vi "Save file.vi"(0 "S1_Current":dbl[](array[numeric]), 1 "S1_Voltage":dbl[](array[numeric]), 2 "S2_Current":dbl[](array[numeric]), 3 "S2_Voltage":dbl[](array[numeric]), 4 "current time":timestamp, 5 "Save path":path, 6 "Save":bool) -> ()   [LabVIEW 2018]
uses:
  <vilib>/Utility/file.llb/Write To Spreadsheet File (string).vi
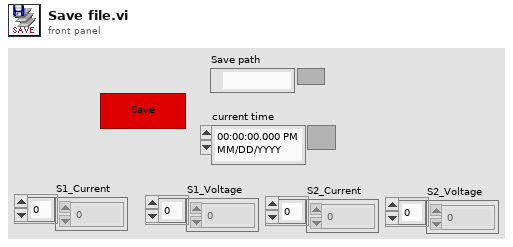
[diagram p1: front panel]
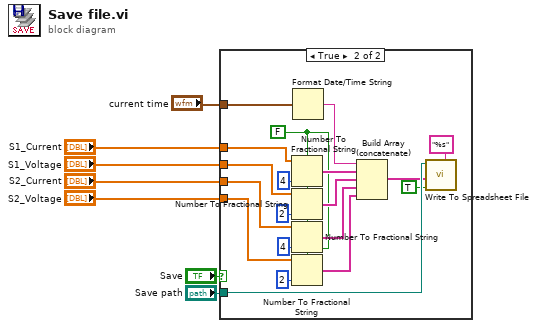
[diagram p0: block diagram]
diagram:
  n1 = case shown="True" "Save" {
    tunnel: "current time" -> [_ w25]
    tunnel: "Save path" -> [_ w12]
    tunnel: "S1_Current" -> [_ w22]
    tunnel: "S1_Voltage" -> [_ w19]
    tunnel: "S2_Current" -> [_ w16]
    tunnel: "S2_Voltage" -> [_ w15]
    frame False {
    }
    frame True {
      w10 = FALSE ("use system decimal point (T)")
      n2 = Number To Fractional String(use system decimal point (T)=w10, number=w22, precision (6)=4) -> (F-format string=w21:string[])  [unwired: 1 in]
      n3 = Number To Fractional String(use system decimal point (T)=w10, number=w19, precision (6)=2) -> (F-format string=w20:string[])  [unwired: 1 in]
      n4 = Number To Fractional String(use system decimal point (T)=w10, number=w16, precision (6)=4) -> (F-format string=w14:string[])  [unwired: 1 in]
      n5 = Number To Fractional String(use system decimal point (T)=w10, number=w15, precision (6)=2) -> (F-format string=w13:string[])  [unwired: 1 in]
      n6 = Format Date/Time String(seconds (now)=w25) -> (date/time string=w26:string)  [unwired: 2 in]
      n7 = Build Array (concatenate)(w26, w21, w20, w14, w13) -> (w11:string[])
      n8 = call-poly <vilib>:"Write To Spreadsheet File.vi"("format (%s)"="%s", "append to file? (new file:F)"=TRUE, "1D data"=w11, "file path (dialog if empty)"=w12) -> ()  [unwired: 4 in, 1 out]
    }
  }
